vi "SigProc_subVI smoothMovAvg.vi"(6 "Size":i32=1 min=1 max=100000, 11 "Signal in":waveform(sgl)) -> (3 "Signal out":waveform(sgl))   [LabVIEW 2018, in "Sig2MS.lvclass"]
uses:
  Sig2MS.lvclass
  <vilib>/Analysis/baseanly.llb/Mean (DBL).vi
  <vilib>/Analysis/NI_AALBase.lvlib
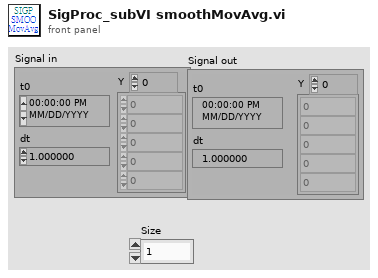
[diagram p1: front panel]
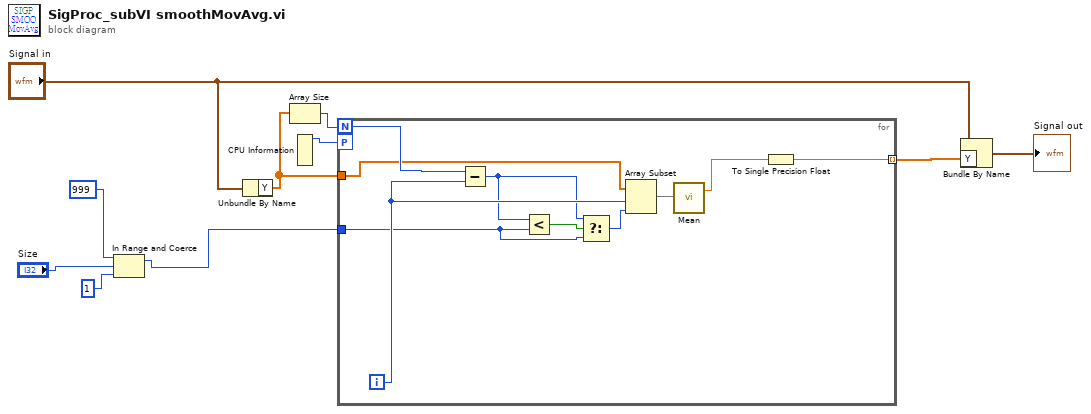
[diagram p0: block diagram]
diagram:
  n1 = In Range and Coerce(upper limit=999, x="Size", lower limit=1) -> (coerced(x)=w7:i32)  [unwired: 1 out]
  n2 = Unbundle By Name("Signal in") -> ("Y"=w5:sgl[])
  n3 = Array Size(array=w5) -> (size(s)=w6:i32)
  n4 = CPU Information() -> (4:w1:i32)  [unwired: 3 out]
  n5 = for {
    N: w6 -> [w20]
    tunnel: w7 -> [w17]
    tunnel: w5 -> [w18]
    tunnel: [w11] -> w4 mode=indexing
    workers-P: w1 -> [_]
    i -> [w19]
    n6 = Subtract(x=w20, y=w19) -> (x-y=w14:i32)
    n7 = Less?(x=w14, y=w17) -> (x < y?=w15:bool)
    n8 = Select(t=w14, s=w15, f=w17) -> (s? t:f=w16:i32)
    n9 = Array Subset(array=w18, index=w19, length=w16) -> (w13:sgl[])
    n10 = call-poly <vilib>:"Mean.vi"("X"=w13) -> ("mean"=w12:dbl)  [unwired: 1 out]
    n11 = To Single Precision Float(number=w12) -> (single precision float=w11:sgl)
  }
  n12 = Bundle By Name(cluster="Signal in", "Y"=w4) -> (→"Signal out":waveform(sgl))
